vi "Window Picker Double Click Detect.vi"(9 "Index (mouse down)":T1, 11 "Loop data (previous)":cluster{"timestamp":dbl, "Index":T1}={"timestamp"=0.0, "Index"={"Row"=-1, "Column"=-1}}) -> (1 "Double Clicked?":bool, 3 "Loop data (new)":cluster{"timestamp":dbl, "Index":T1}={"timestamp"=0.0, "Index"={"Row"=-1, "Column"=-1}})   [LabVIEW 2021, in "MultiStokePlot.lvlib" / "MultiPlotPanel.lvclass"]
uses:
  Classes/MultiPlotPanel/MultiPlotPanel.lvclass
  <vilib>/Utility/miscctls.llb/LVRowAndColumnTypeDef.ctl
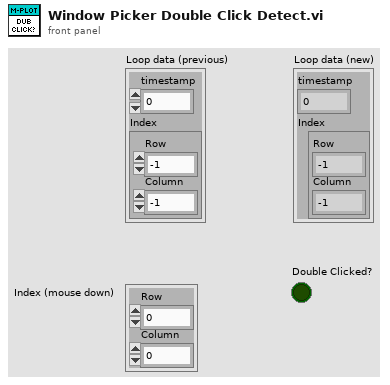
[diagram p1: front panel]
types:
  T1 = typedef "LVRowAndColumnTypeDef.ctl" = cluster{"Row":i32, "Column":i32}
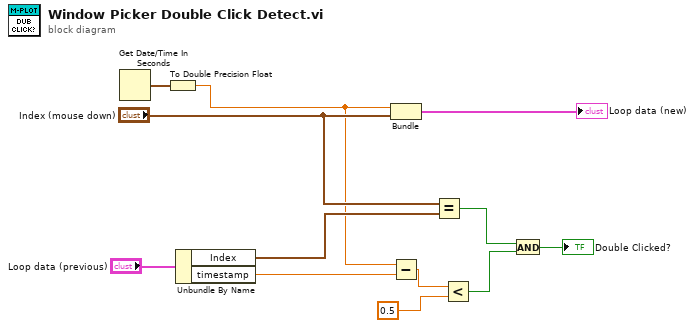
[diagram p0: block diagram]
diagram:
  n1 = Get Date/Time In Seconds() -> (seconds since 1Jan1904=w12:timestamp)
  n2 = To Double Precision Float(number=w12) -> (double precision float=w7:dbl)
  n3 = Unbundle By Name("Loop data (previous)") -> ("Index"=w8:T1, "timestamp"=w6:dbl)
  n4 = Bundle(w7, "Index (mouse down)"="Index (mouse down)") -> (→"Loop data (new)":cluster{dbl, "Index (mouse down)":T1})  [unwired: 1 in]
  n5 = Subtract(x=w7, y=w6) -> (x-y=w5:dbl)
  n6 = Equal?(x="Index (mouse down)", y=w8) -> (x = y?=w2:bool)
  n7 = Less?(x=w5, y=0.5) -> (x < y?=w3:bool)
  n8 = And(x=w2, y=w3) -> (x .and. y?=→"Double Clicked?":bool)
